vi "Set Out.vi"(8 "error in (no error)":errorcluster, 10 "Output value":refnum<class "Output Value.lvclass">, 11 "Oxford PS Driver in":refnum<class "Oxford PS Driver.lvclass">) -> (0 "error out":errorcluster, 3 "Oxford PS Driver out":refnum<class "Oxford PS Driver.lvclass">)   [LabVIEW 2018, in "Oxford PS Driver.lvclass"]
uses:
  Oxford PS Driver.lvclass
  C:/github/NHMFL_Core/Libraries/Instruments/VISA Instrument/VISA Instrument.lvclass
  Utilities/Output Value/Output Value.lvclass
  C:/github/NHMFL_Core/Libraries/Instruments/Results/Acquired Result/Acquired Result.lvclass
  VISA Instrument/VISA Instrument.lvclass/VISA Instrument.ctl
  VISA Instrument/Read VISA resource.vi
  VISA Instrument/Write VISA resource.vi
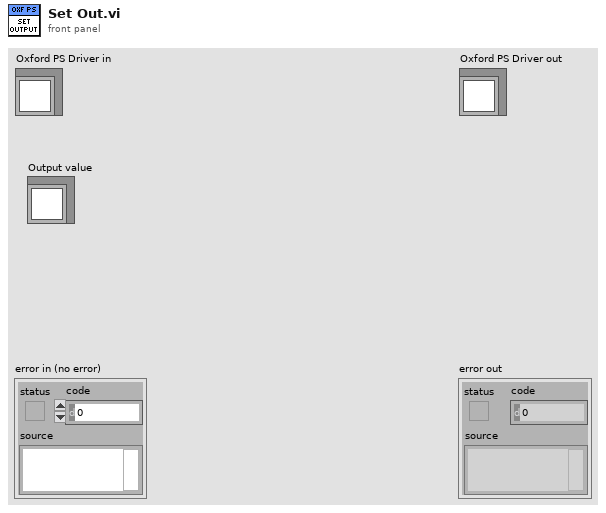
[diagram p1: front panel]
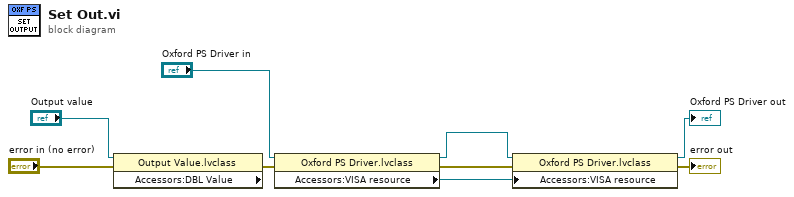
[diagram p0: block diagram]
diagram:
  n1 = property class="Output Value.lvclass" props=["Accessors:DBL Value"](reference="Output value", error in="error in (no error)") -> (error out=w8:errorcluster)  [unwired: 2 out]
  n2 = property class="Oxford PS Driver.lvclass"(reference="Oxford PS Driver in", error in=w8) -> (reference out=w7:refnum<class "Oxford PS Driver.lvclass">, error out=w9:errorcluster, "Accessors:VISA resource"=w6:refnum<visa-resource-name>)
  n3 = property class="Oxford PS Driver.lvclass"(reference=w7, error in=w9, "Accessors:VISA resource"=w6) -> (reference out=→"Oxford PS Driver out":refnum<class "Oxford PS Driver.lvclass">, error out=→"error out":errorcluster)
